vi "init_ControlsSD.vi"() -> (2 "Controls":T1, 3 "error out":errorcluster)   [LabVIEW 2015]
uses:
  controls/Controls.ctl
  Classes/Experiment.lvclass
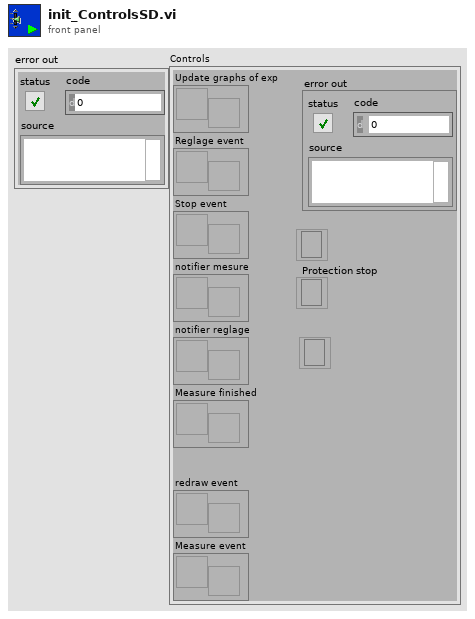
[diagram p1: front panel]
types:
  T1 = typedef "Controls.ctl" = cluster{"Update graphs of exp":refnum<user-event>, "Reglage event":refnum<user-event>, "Stop event":refnum<user-event>, "notifier mesure":refnum<notifier>, "notifier reglage":refnum<notifier>, "Measure finished":refnum<user-event>, "control registration ref":refnum<event-registration>, "redraw event":refnum<user-event>, "Measure event":refnum<user-event>, "Mes, Reg, Stop Registration ref":refnum<event-registration>, "error out":errorcluster, "Protection stop":refnum<event-registration>}
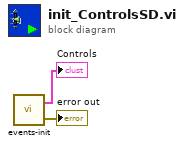
[diagram p0: block diagram]
diagram:
  n1 = call "events-init.vi"() -> ("sortie d'erreur"=→"error out":errorcluster, "Controls"=→"Controls":T1)  [unwired: 2 in]
